vi "Eliminated.vi"(6 "Column":i32, 8 "Row":i32, 9 "Killer":i32, 10 "Team":i32, 11 "Template in":refnum<class "Demo.lvclass">) -> (3 "Template out":refnum<class "Demo.lvclass">)   [LabVIEW 2020, in "Demo.lvclass"]
uses:
  Demo.lvclass
  Square/Square.lvclass
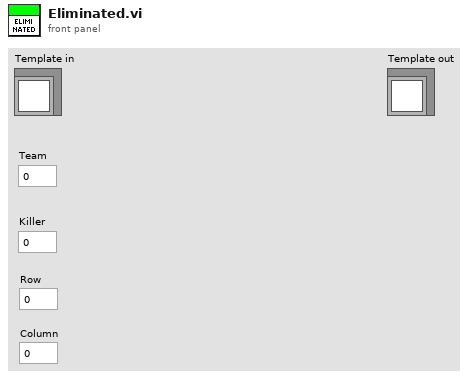
[diagram p1: front panel]
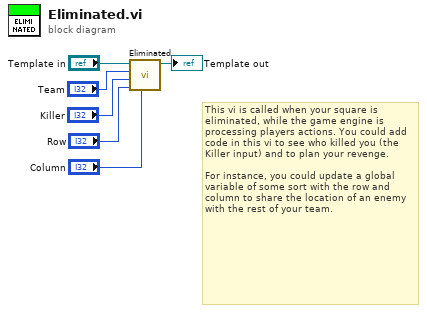
[diagram p0: block diagram]
diagram:
  # "This vi is called when your square is eliminated, while the game engine is processing players actions. You could add code in this vi to see who killed you (the Killer input) and to plan your revenge. \n\nFor instance, you could update a global variable of some sort with the row and column to share the location of an enemy with the rest of your team."
  n1 = call-parent "Eliminated.vi"("Column"="Column", "Row"="Row", "Killer Index"="Killer", "Team Index"="Team", "Square in"="Template in") -> ("Square out"=→"Template out":refnum<class "Demo.lvclass">)  [unwired: 6 in]
